vi "Write Calling VI Name.vi"(10 "Calling VI Name":string, 11 "Show Assert in":refnum<class "Show Assert.lvclass">) -> (3 "Show Assert out":refnum<class "Show Assert.lvclass">)   [LabVIEW 2018, in "Assert API Components.lvlib" / "Assert Display.lvlib" / "Main Display.lvlib" / "Show Assert.lvclass"]
uses:
  Show Assert.lvclass
  Show Assert.lvclass/Show Assert.ctl
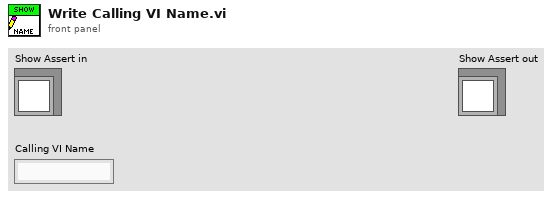
[diagram p1: front panel]
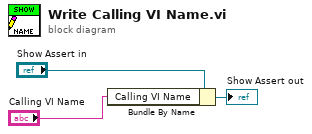
[diagram p0: block diagram]
diagram:
  n1 = Bundle By Name(cluster="Show Assert in", "Calling VI Name"="Calling VI Name") -> (→"Show Assert out":refnum<class "Show Assert.lvclass">)
